vi "HTML Report Numeric Tag Attribute.vi"(4 "default value (0)":i32, 5 "value":i32, 6 "label":string, 7 "tag attributes in":string) -> (3 "tag attributes out":string)   [LabVIEW 2020, in "NI_ReportGenerationCore.lvlib"]
doc: "For non-default value, constructs the appropriate attribute."
uses:
  <vilib>/Utility/NIReport.llb/NI_ReportGenerationCore.lvlib
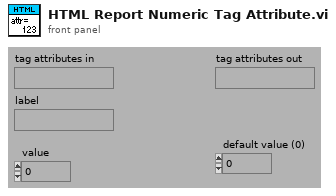
[diagram p1: front panel]
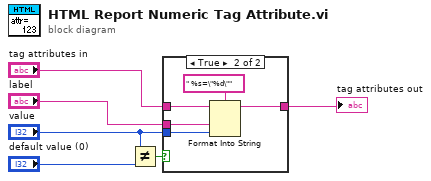
[diagram p0: block diagram]
diagram:
  n1 = Not Equal?(x="value", y="default value (0)") -> (x != y?=w1:bool)
  n2 = case shown="True" w1 {
    tunnel: [w7 w12] -> w4
    tunnel: "tag attributes in" -> [w7 w11]
    tunnel: "value" -> [_ w9]
    tunnel: "label" -> [_ w8]
    frame False {
    }
    frame True {
      n3 = Format Into String(format string=" %s=\"%d\"", initial string=w11, w8, w9) -> (resulting string=w12:string)  [unwired: 1 in, 1 out]
    }
  }
  "tag attributes out" <- w4
